vi "Test.vi"   [LabVIEW 2012]
doc: "This VI is called when test mode begins, and will automatically be terminated when it ends. You can add manual or automatic tests and invoke them from the dashboard."
uses:
  <vilib>/Rock Robotics/SystemInterfaces/Typedef/FPGA_TypedefDigitalModule.ctl
  <vilib>/Rock Robotics/SystemInterfaces/DIO/FPGA_DIOChannel.ctl
  <vilib>/Rock Robotics/SystemInterfaces/DIO/FPGA_DIORelayChannel.ctl
  Robot Global Data.vi
  <vilib>/Rock Robotics/WPI/Compressor/WPI_CompressorGetSetRefNum.vi
types:
  T1 = typedef "FPGA_DIORelayChannel.ctl" = enum8{"Relay 1", "Relay 2", "Relay 3", "Relay 4", "Relay 5", "Relay 6", "Relay 7", "Relay 8", "Invalid"}
  T2 = typedef "FPGA_DIOChannel.ctl" = enum8{"DIO 1", "DIO 2", "DIO 3", "DIO 4", "DIO 5", "DIO 6", "DIO 7", "DIO 8", "DIO 9", "DIO 10", "DIO 11", "DIO 12", "DIO 13", "DIO 14", "Invalid"}
  T3 = typedef "FPGA_TypedefDigitalModule.ctl" = enum16{"Digital Module 1", "Digital Module 2"}
  T4 = typedef "WPI_CompressorDevRef.ctl" = cluster{"DevStatus":errorcluster, "DigitalInputDevRef":T5, "RelayDevRef":T6}
  T5 = typedef "WPI_DigitalInputDevRef.ctl" = cluster{"DevStatus":errorcluster, "DIO Channel":T2, "Digital Module":T3}
  T6 = typedef "WPI_RelayDevRef.ctl" = cluster{"DevStatus":errorcluster, "Relay Channel":T1, "Digital Module":T3, "Relay Direction":T7}
  T7 = typedef "WPI_RelayDirection.ctl" = enum16{"Both directions", "Forward only", "Reverse only"}
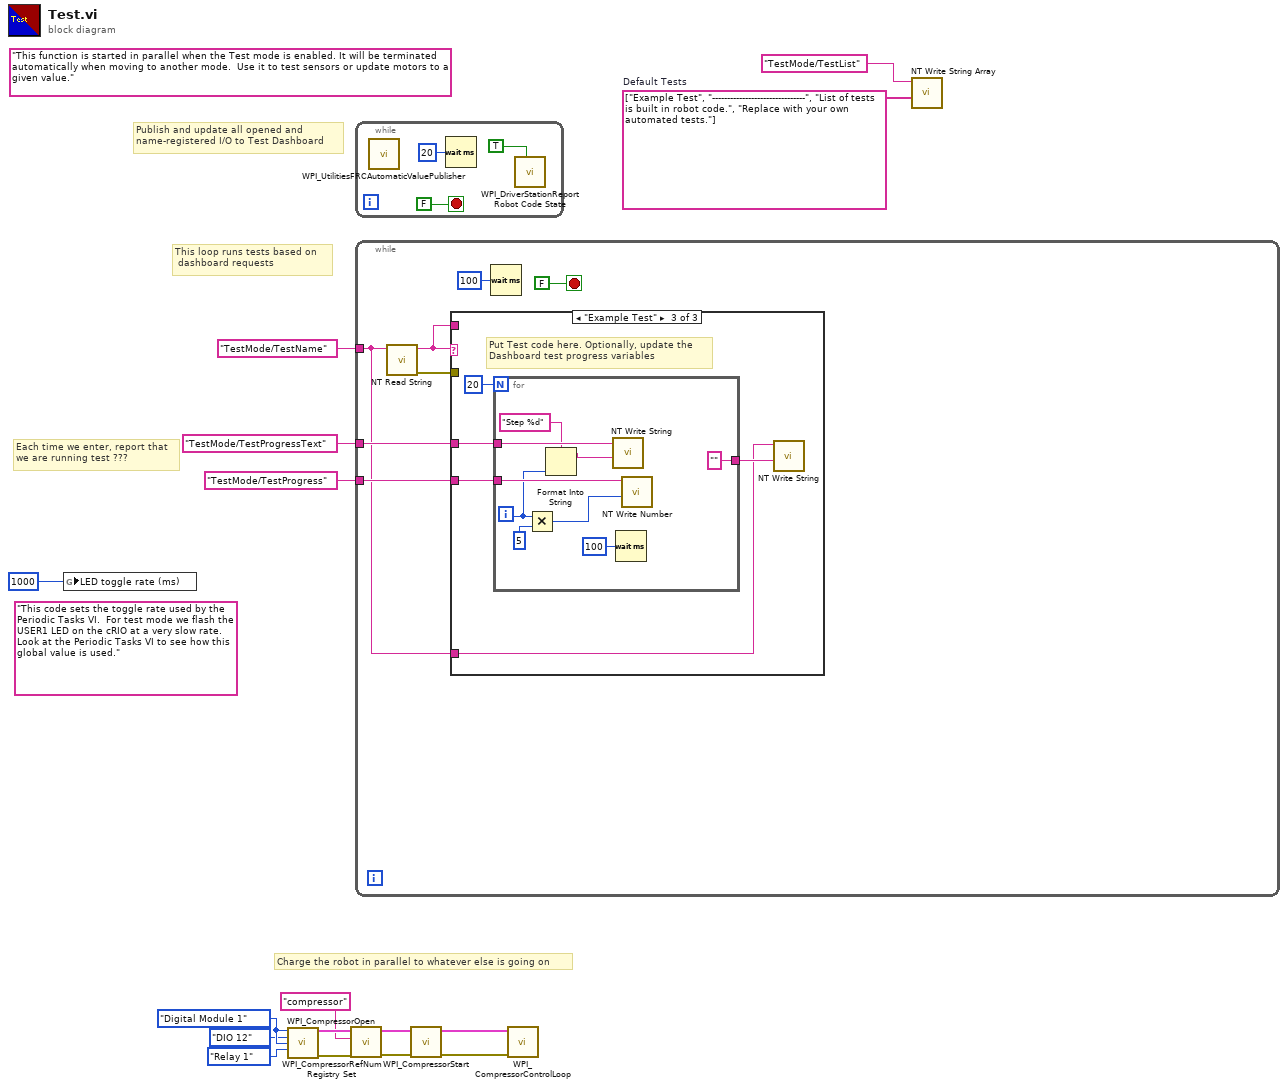
[diagram p0: block diagram]
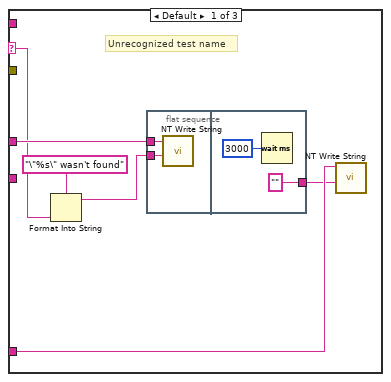
[diagram p2: hidden frame]
diagram:
  w9 = FPGA_TypedefDigitalModule."Digital Module 1" ("Pressure Switch Digital Module (Module 1)")
  w12 = string[] ["Example Test", "-------------------------------", "List of tests is built in robot code.", "Replace with your own automated tests."]  # Default Tests
  (unwired) "This code sets the toggle rate used by the Periodic Tasks VI.  For test mode we flash the USER1 LED on the cRIO at a very slow rate.  Look at the Periodic Tasks VI to see how this global value is used."
  (unwired) "This function is started in parallel when the Test mode is enabled. It will be terminated automatically when moving to another mode.  Use it to test sensors or update motors to a given value."
  # "Charge the robot in parallel to whatever else is going on"
  # "This loop runs tests based on \n dashboard requests"
  # "Publish and update all opened and\nname-registered I/O to Test Dashboard"
  # "Each time we enter, report that\nwe are running test ???"
  n1 = global write "Robot Global Data.vi" "LED toggle rate (ms)"(u32 1000 ("LED ms toggle rate")) -> ()
  n2 = call <vilib>:"WPI_CompressorOpen.vi"("Pressure Switch Digital Module (Module 1)"=w9, "Pressure Switch DIO Channel"=FPGA_DIOChannel."DIO 12", "Relay Digital Module (Module 1)"=w9, "Relay Channel"=FPGA_DIORelayChannel."Relay 1") -> ("CompressorDevRef"=w6:T4, "error out"=w7:errorcluster)  [unwired: 10 in]
  n3 = call <vilib>:"WPI_CompressorRefNum Registry Set.vi"("error in (no error)"=w7, "refnum name"="compressor", "CompressorDevRef"=w6) -> ("error out"=w4:errorcluster, "CompressorDevRef"=w5:T4)  [unwired: 7 in]
  n4 = while {
    stop <- FALSE stop-if-true
    n5 = call <vilib>:"WPI_UtilitiesFRCAutomaticValuePublisher.vi"() -> ()  [unwired: 12 in]
    n6 = Wait (ms)(milliseconds to wait=u32 20) -> ()  [unwired: 1 out]
    n7 = call <vilib>:"WPI_DriverStationReport Robot Code State.vi"("Test"=TRUE ("Autonomous")) -> ()  [unwired: 10 in, 1 out]
  }
  n8 = while {
    tunnel: "TestMode/TestName" ("Name") -> [w21]
    tunnel: "TestMode/TestProgressText" ("Name") -> [w24]
    tunnel: "TestMode/TestProgress" ("Name") -> [w23]
    stop <- FALSE stop-if-true
    n9 = call <vilib>:"NT Read String.vi"("Name"=w21) -> ("error out"=w20:errorcluster, "String"=w22:string)  [unwired: 9 in]
    n10 = case shown="\"Example Test\"" w22 {
      selector: w22 -> [w31 _ _]
      tunnel: w21 -> [w28 _ w37]
      tunnel: w24 -> [w32 _ w40]
      tunnel: w23 -> [_ _ w41]
      tunnel: w22 -> [_ _ _]
      tunnel: w20 -> [_ _ _]
      frame Default {
        # "Unrecognized test name"
        n11 = Format Into String(format string="\"%s\" wasn't found" ("Name"), w31) -> (resulting string=w30:string)  [unwired: 2 in, 1 out]
        n12 = flat-sequence {
          tunnel: w32 -> [w33]
          tunnel: w30 -> [w34]
          tunnel: ["" ("Name")] -> w27
          frame #0 {
            n13 = call <vilib>:"NT Write String.vi"("String"=w34, "Name"=w33) -> ()  [unwired: 9 in, 1 out]
          }
          frame #1 {
            n14 = Wait (ms)(milliseconds to wait=u32 3000) -> ()  [unwired: 1 out]
          }
        }
        n15 = call <vilib>:"NT Write String.vi"("String"=w27, "Name"=w28) -> ()  [unwired: 9 in, 1 out]
      }
      frame "" {
        # "No test to run"
      }
      frame "Example Test" {
        # "Put Test code here. Optionally, update the\nDashboard test progress variables"
        n16 = for {
          N: 20 -> [_]
          tunnel: w41 -> [w50]
          tunnel: w40 -> [w48]
          tunnel: ["" ("String")] -> w38
          i -> [w45]
          n17 = Multiply(x=w45, y=u32 5 ("milliseconds to wait")) -> (x*y=w46:u32)
          n18 = Format Into String(format string="Step %d", w45) -> (resulting string=w43:string)  [unwired: 2 in, 1 out]
          n19 = call <vilib>:"NT Write String.vi"("String"=w43, "Name"=w48) -> ()  [unwired: 9 in, 1 out]
          n20 = Wait (ms)(milliseconds to wait=u32 100) -> ()  [unwired: 1 out]
          n21 = call <vilib>:"NT Write Number.vi"("Numeric"=w46, "Name"=w50) -> ()  [unwired: 9 in, 1 out]
        }
        n22 = call <vilib>:"NT Write String.vi"("String"=w38, "Name"=w37) -> ()  [unwired: 9 in, 1 out]
      }
    }
    n23 = Wait (ms)(milliseconds to wait=u32 100) -> ()  [unwired: 1 out]
  }
  n24 = call <vilib>:"WPI_CompressorStart.vi"("error in (no error)"=w4, "CompressorDevRef"=w5) -> ("error out"=w2:errorcluster, "CompressorDevRef"=w1:T4)  [unwired: 8 in]
  n25 = call <vilib>:"WPI_CompressorControlLoop.vi"("error in (no error)"=w2, "CompressorDevRef"=w1) -> ()  [unwired: 10 in]
  n26 = call <vilib>:"NT Write String Array.vi"("String Array"=w12, "Name"="TestMode/TestList") -> ()  [unwired: 9 in, 1 out]
